vi "EquationEditor.vi"(0 "VISA IN":refnum<visa-resource-name>, 5 "error in":errorcluster, 6 "Equation or Expression":string, 7 "Channel":i32=1, 11 "EqOn-Off":bool) -> (14 "VISA Out":refnum<visa-resource-name>, 19 "error out":errorcluster)   [LabVIEW 2018, in "PNA-X.lvlib"]
uses:
  PNA-X.lvlib
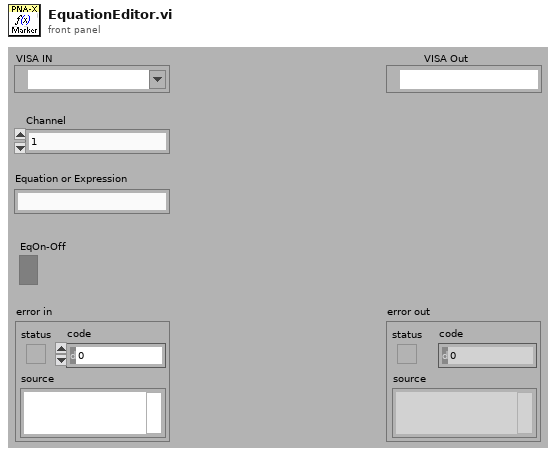
[diagram p1: front panel]
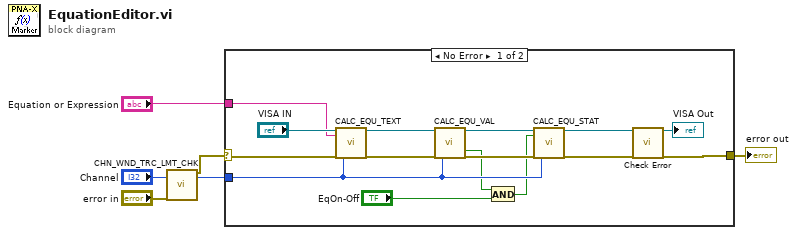
[diagram p0: block diagram]
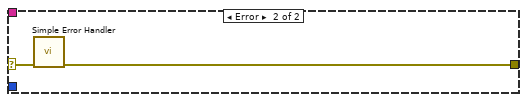
[diagram p2: hidden frame]
diagram:
  n1 = call "CHN_WND_TRC_LMT_CHK.vi"("Channel"="Channel", "error in"="error in") -> ("error out"=w2:errorcluster, "Channel"=w1:i32)  [unwired: 13 in, 3 out]
  n2 = case shown="No Error" w2 {
    selector: w2 -> [w19 w23]
    tunnel: [w21 w22] -> w5
    tunnel: "Equation or Expression" -> [w11 _]
    tunnel: w1 -> [w10 _]
    frame No Error {
      n3 = call "CALC_EQU_TEXT.vi"("VISA IN"="VISA IN", "Equation or Expression"=w11, "error in"=w19, "Channel"=w10) -> ("VISA Out"=w14:refnum<visa-resource-name>, "error out"=w18:errorcluster)  [unwired: 14 in]
      n4 = call "CALC_EQU_VAL.vi"("VISA IN"=w14, "error in"=w18, "Channel"=w10) -> ("VISA Out"=w13:refnum<visa-resource-name>, "EqValid?"=w9:bool, "error out"=w17:errorcluster)  [unwired: 14 in]
      n5 = And(x=w9, y="EqOn-Off") -> (x .and. y?=w7:bool)
      n6 = call "CALC_EQU_STAT.vi"("VISA IN"=w13, "Equation ON/OFF"=w7, "error in"=w17, "Channel"=w10) -> ("VISA Out"=w12:refnum<visa-resource-name>, "error out"=w16:errorcluster)  [unwired: 14 in]
      n7 = call "Check Error.vi"("VISA Resource Name"=w12, "error in (no error)"=w16) -> ("dup VISA session"=→"VISA Out":refnum<visa-resource-name>, "error out"=w21:errorcluster)  [unwired: 16 in]
    }
    frame Error {
      n8 = call <vilib>:"Simple Error Handler.vi"("error in (no error)"=w23) -> ("error out"=w22:errorcluster)  [unwired: 4 in, 4 out]
    }
  }
  "error out" <- w5
